vi "Enqueue Msg.vi"(8 "error in (no error)":errorcluster, 9 "Data":variant, 10 "Message":string, 11 "Queue in":refnum<queue>) -> (0 "error out":errorcluster, 3 "Queue out":refnum<queue>)   [LabVIEW 2020]
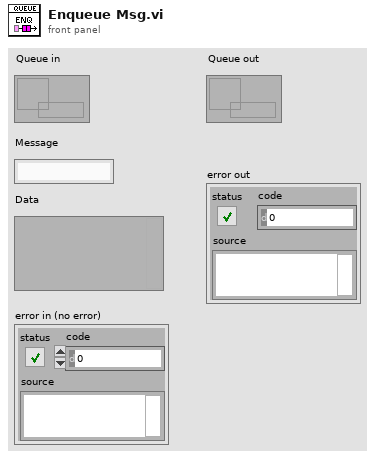
[diagram p1: front panel]
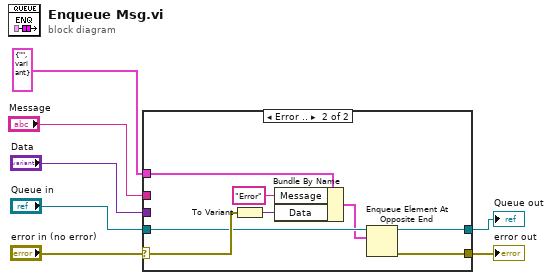
[diagram p0: block diagram]
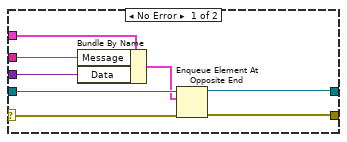
[diagram p2: hidden frame]
diagram:
  n1 = case shown="Error .." "error in (no error)" {
    selector: "error in (no error)" -> [w13 w22]
    tunnel: [w12 w19] -> w5
    tunnel: "Queue in" -> [w15 w21]
    tunnel: [w14 w20] -> w7
    tunnel: "Message" -> [w10 _]
    tunnel: "Data" -> [w9 _]
    tunnel: cluster{"Message":string, "Data":variant} {"Message"="", "Data"=variant} ("element") -> [w8 w17]
    frame No Error {
      n2 = Bundle By Name(cluster=w8, "Message"=w10, "Data"=w9) -> (w11:cluster{"Message":string, "Data":variant})
      n3 = Enqueue Element At Opposite End(queue=w15, element=w11, error in (no error)=w13) -> (queue out=w14:refnum<queue>, error out=w12:errorcluster)  [unwired: 1 in, 1 out]
    }
    frame Error {
      n4 = To Variant(anything=w22) -> (Variant=w23:variant)
      n5 = Bundle By Name(cluster=w17, "Message"="Error", "Data"=w23) -> (w18:cluster{"Message":string, "Data":variant})
      n6 = Enqueue Element At Opposite End(queue=w21, element=w18) -> (queue out=w20:refnum<queue>, error out=w19:errorcluster)  [unwired: 2 in, 1 out]
    }
  }
  "Queue out" <- w7
  "error out" <- w5
